vi "formatTemptoXML.vi"() -> ()   [LabVIEW 2019]
panel:
  in  "Array":dbl[][][][][][][][](array[numeric])
  out "error out":errorcluster
  out "Temprature Charts":dbl[](graph)
  out "Numeric":dbl
  in  "Thermometer":dbl(slide) scale=0.0..100.0
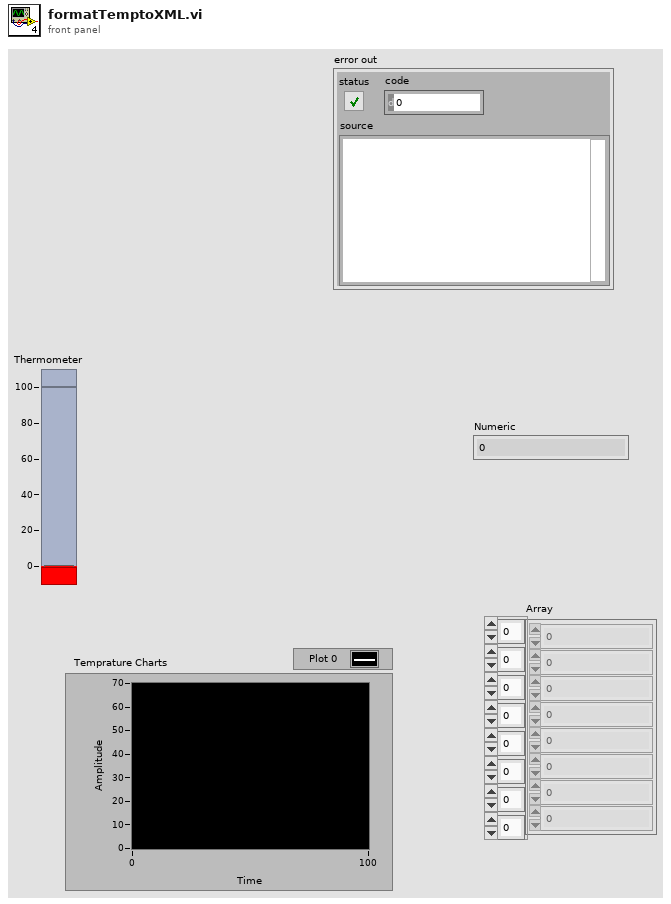
[diagram p1: front panel]
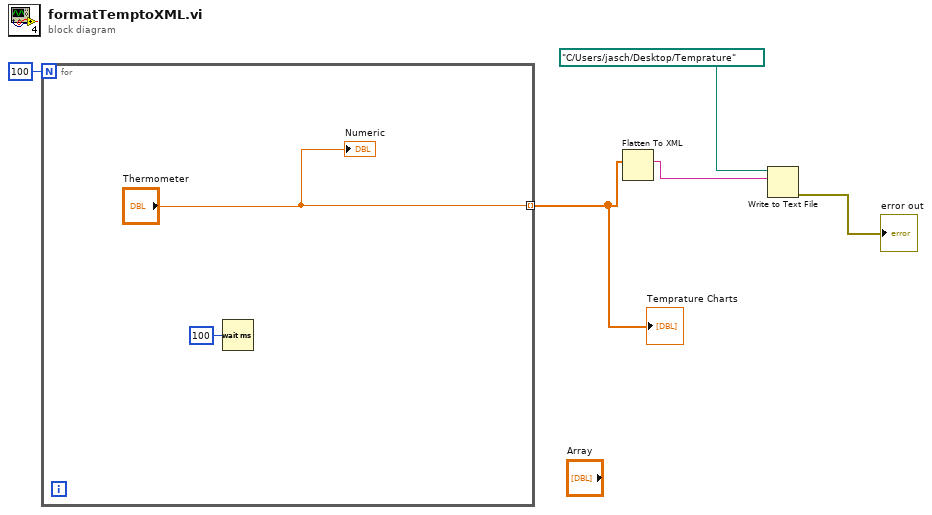
[diagram p0: block diagram]
diagram:
  n1 = for {
    N: 100 -> [_]
    tunnel: ["Thermometer"] -> w4 mode=indexing
    n2 = Wait (ms)(milliseconds to wait=u32 100) -> ()  [unwired: 1 out]
    "Numeric" <- "Thermometer"
  }
  "Temprature Charts" <- w4
  n3 = Flatten To XML(anything=w4) -> (xml string=w2:string)
  n4 = Write to Text File(file (use dialog)=path "C:/Users/jasch/Desktop/Temprature", text=w2) -> (error out=→"error out":errorcluster)  [unwired: 2 in, 2 out]
